vi "SP - click on ctrl.vi"(7 "Control Label":string, 8 "error in (no error)":errorcluster, 10 "subVI":refnum<vi>, 11 "VI with Focus":refnum<vi>) -> (0 "error out":errorcluster, 3 "return value":string)   [LabVIEW 2020, in "ui-testing.lvlib"]
uses:
  ui-testing.lvlib
  User32.dll
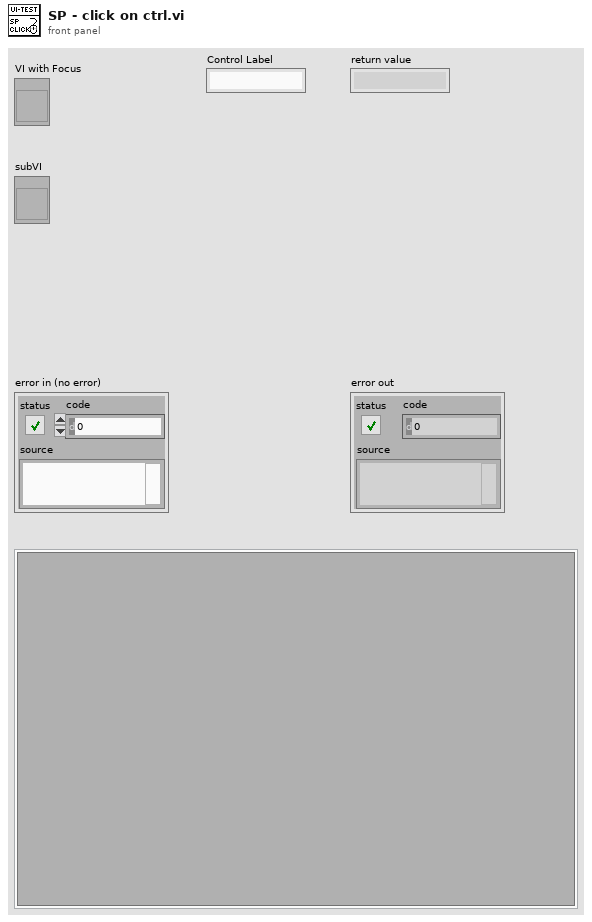
[diagram p1: front panel]
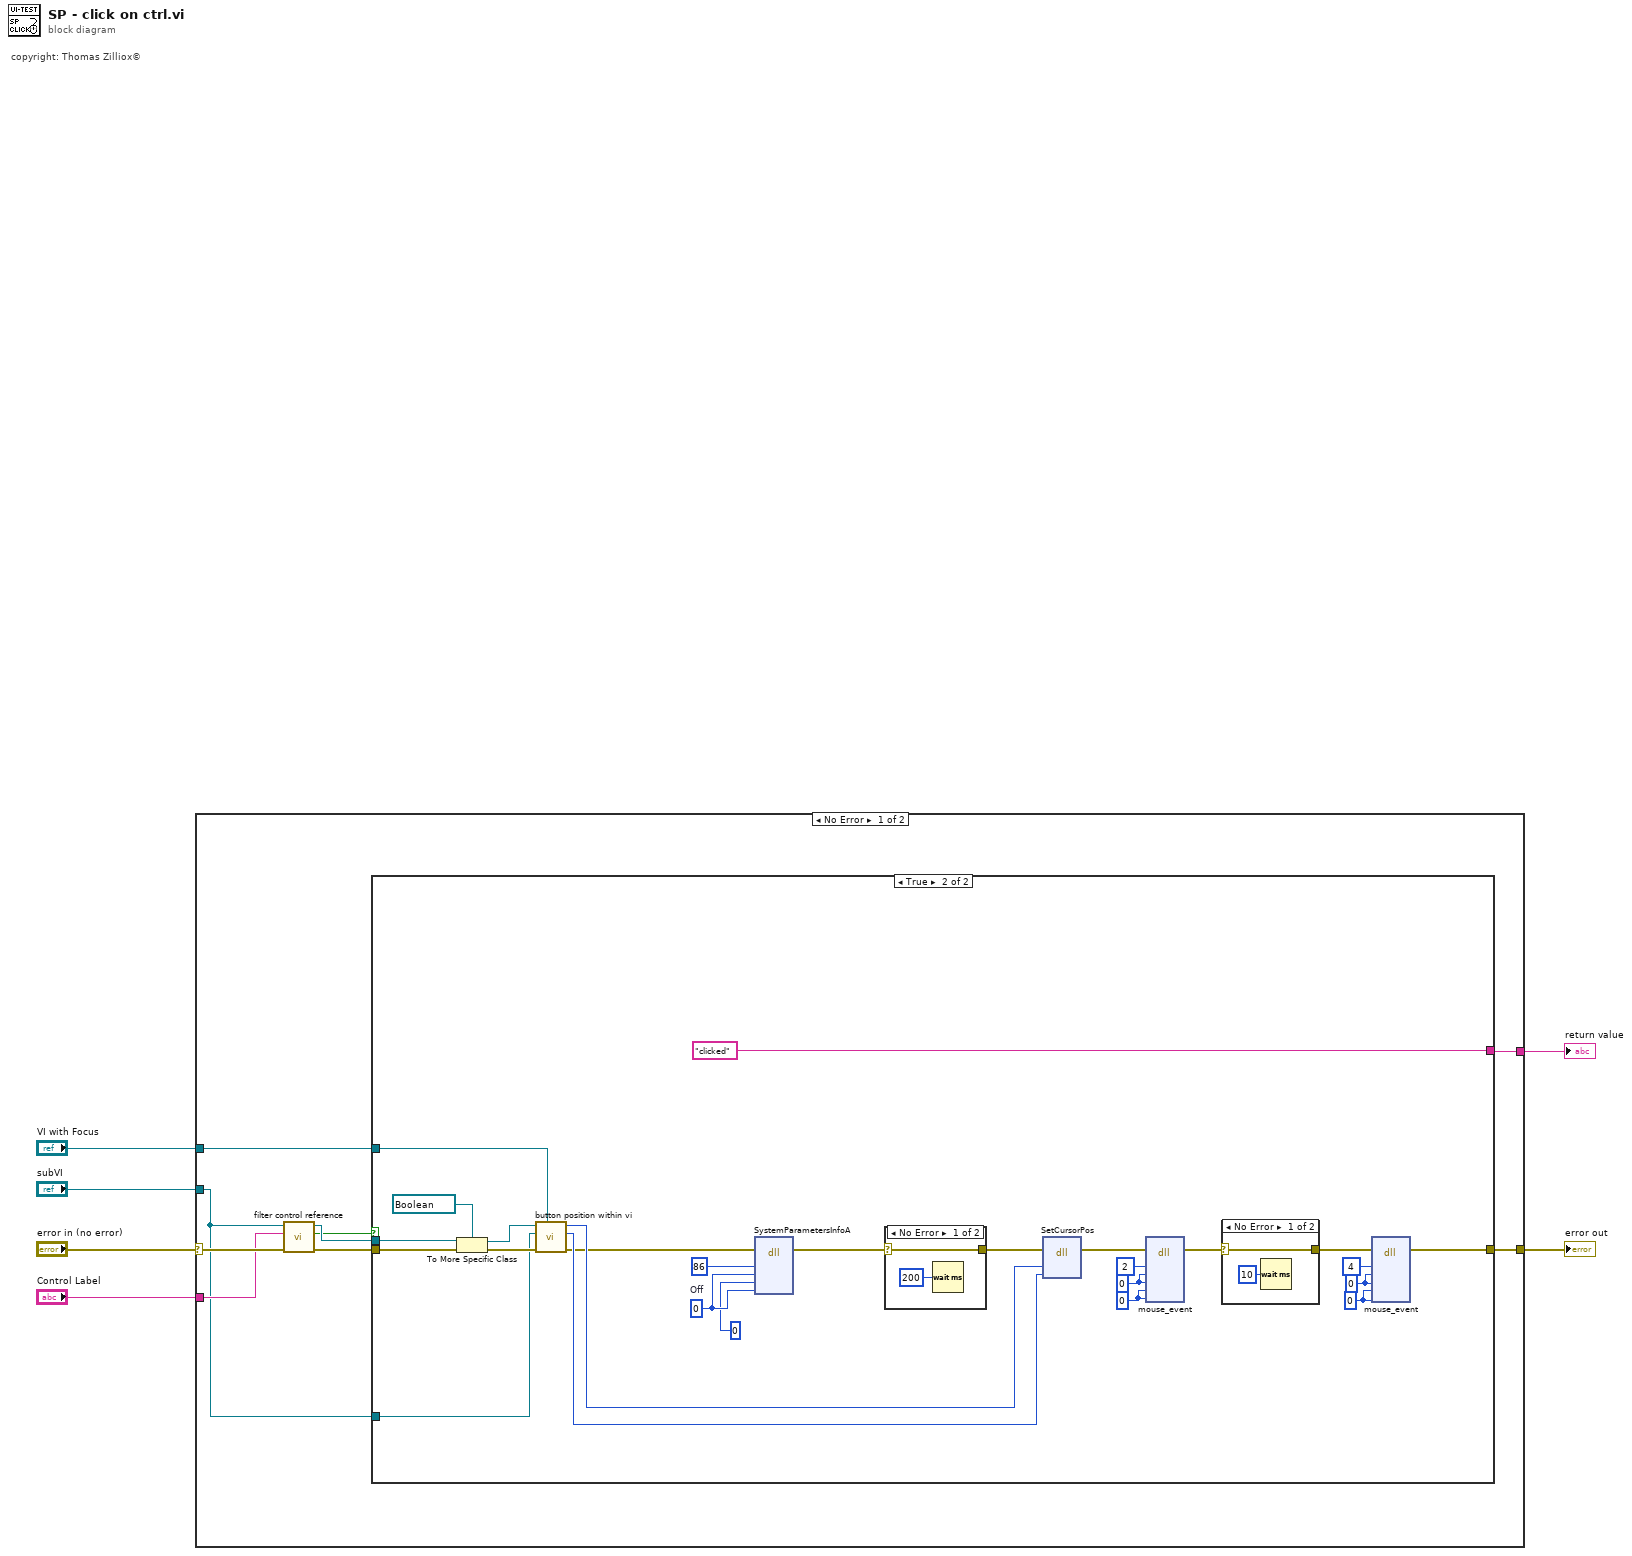
[diagram p0: block diagram]
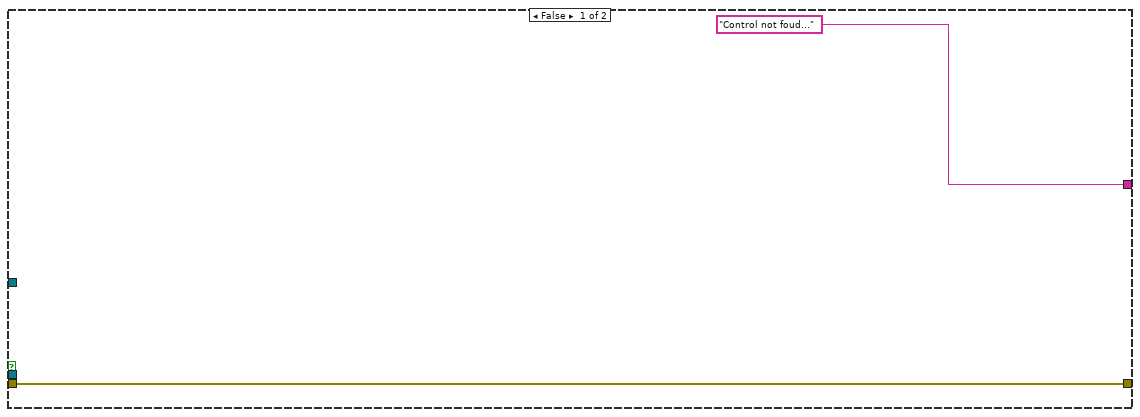
[diagram p2: hidden frame]
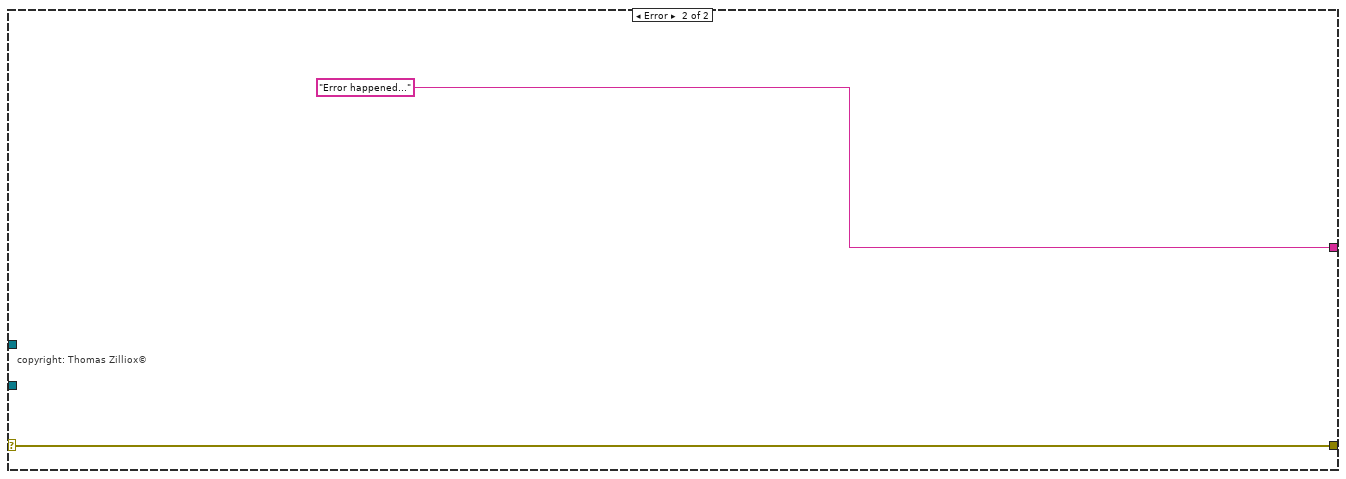
[diagram p5: hidden frame]
diagram:
  # "copyright: Thomas Zilliox©"
  n1 = case shown="No Error" "error in (no error)" {
    selector: "error in (no error)" -> [w12 w51]
    tunnel: [w13 w51] -> w5
    tunnel: "Control Label" -> [w10 _]
    tunnel: [w14 "Error happened..."] -> w3
    tunnel: "subVI" -> [w8 _]
    tunnel: "VI with Focus" -> [w11 _]
    frame No Error {
      n2 = call "filter control reference.vi"("error in (no error)"=w12, "Control label"=w10, "VI (Caller)"=w8) -> ("error out"=w7:errorcluster, "Control found"=w9:bool, "Control ref"=w15:refnum<vi>)  [unwired: 6 in]
      n3 = case shown="True" w9 {
        tunnel: w15 -> [_ w43]
        tunnel: w7 -> [w16 w42]
        tunnel: ["Control not foud..." ("VI Name") "clicked" ("VI Name")] -> w14
        tunnel: [w16 w24] -> w13
        tunnel: w11 -> [_ w20]
        tunnel: w8 -> [_ w21]
        frame False {
        }
        frame True {
          w30 = 0 ("dwExtraInfo")
          w31 = u32 0 ("dwExtraInfo")
          w29 = 0 ("dwExtraInfo")
          w28 = u32 0 ("dwExtraInfo")
          w41 = u32 0  # Off
          n4 = To More Specific Class(target class=refnum<vi> refnum ("Boolean in"), reference=w43, error in=w42) -> (specific class reference=w19:refnum<vi>, error out=w23:errorcluster)
          n5 = call "button position within vi.vi"("VI with focus"=w20, "error in (no error)"=w23, "VI Reference"=w21, "Boolean in"=w19) -> ("error out"=w18:errorcluster, "Vertical"=w35:i16, "Horizontal"=w36:i16)  [unwired: 3 in, 2 out]
          n6 = dll-call lib="User32.dll" fn="SystemParametersInfoA" label="Terminate power-off mode"(error in=w18, "uiAction"=u32 86 ("SPI_GETPOWEROFFACTIVE"), "uiParam"=w41, "pvParam"=0, "fWinIni"=w41) -> (error out=w38:errorcluster)  [unwired: 7 in, 1 out]
          n7 = case shown="No Error" w38 {
            selector: w38 -> [w47 w49]
            tunnel: [w47 w49] -> w37
            frame No Error {
              n8 = Wait (ms)(milliseconds to wait=u32 200) -> ()  [unwired: 1 out]
            }
            frame Error {
            }
          }
          n9 = dll-call lib="User32.dll" fn="SetCursorPos" label="Move mouse"(error in=w37, "dx"=w36, "dy"=w35) -> (error out=w33:errorcluster)  [unwired: 5 in, 1 out]
          n10 = dll-call lib="User32.dll" fn="mouse_event" label="Click"(error in=w33, "dwFlags"=2, "dx"=w29, "dy"=w29, "dwData"=w28, "dwExtraInfo"=w28) -> (error out=w26:errorcluster)  [unwired: 8 in, 1 out]
          n11 = case shown="No Error" w26 {
            selector: w26 -> [w44 w46]
            tunnel: [w44 w46] -> w25
            frame No Error {
              n12 = Wait (ms)(milliseconds to wait=u32 10) -> ()  [unwired: 1 out]
            }
            frame Error {
            }
          }
          n13 = dll-call lib="User32.dll" fn="mouse_event" label="Release"(error in=w25, "dwFlags"=4, "dx"=w30, "dy"=w30, "dwData"=w31, "dwExtraInfo"=w31) -> (error out=w24:errorcluster)  [unwired: 8 in, 1 out]
        }
      }
    }
    frame Error {
      # "copyright: Thomas Zilliox©"
    }
  }
  "error out" <- w5
  "return value" <- w3
